vi "Create Reference Maps.vi"(8 "error in (no error)":errorcluster, 10 "RT Target":bool, 11 "LabVIEW Build Script in":refnum<class "LabVIEW Build Script.lvclass">) -> (0 "error out":errorcluster, 3 "LabVIEW Build Script out":refnum<class "LabVIEW Build Script.lvclass">)   [LabVIEW 2021, in "LabVIEW Build Script.lvclass"]
uses:
  LabVIEW Build Script.lvclass
  LabVIEW Build Script.lvclass/LabVIEW Build Script.ctl
  <vilib>/CIF Foundation/CIF LabVIEW Scripting/LV Scripting/LV Scripting Utilities.lvlib
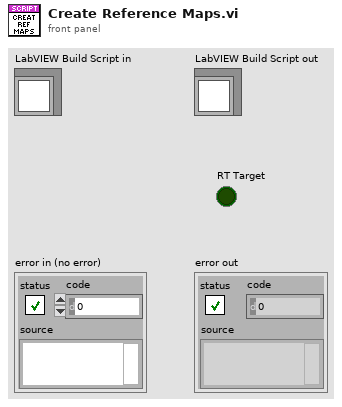
[diagram p1: front panel]
types:
  T1 = typedef "LV Scripting Utilities.lvlib/Target References.ctl" = cluster{"Target Reference":refnum<vi>, "VI References":refnum<vi>[], "Library References":refnum<vi>[], "Build References":refnum<vi>[]}
  T2 = typedef "LV Scripting Utilities.lvlib/BuildSpec Map.ctl" = map{string, refnum<vi>}
  T3 = typedef "LV Scripting Utilities.lvlib/Library Map.ctl" = map{string, refnum<vi>}
  T4 = typedef "LV Scripting Utilities.lvlib/VI Map.ctl" = map{string, refnum<vi>}
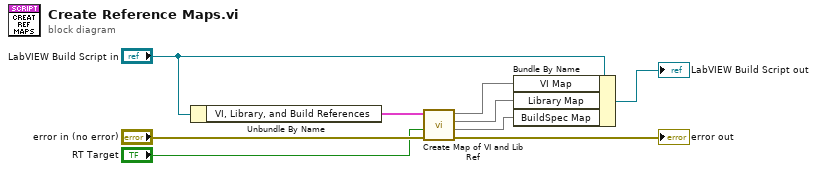
[diagram p0: block diagram]
diagram:
  n1 = Unbundle By Name("LabVIEW Build Script in") -> ("VI, Library, and Build References"=w7:T1[])
  n2 = call <vilib>:"Create Map of VI and Lib Ref.vi"("error in"="error in (no error)", "RT Target"="RT Target", "VI, Library, and Build References"=w7) -> ("error out"=→"error out":errorcluster, "BuildSpec Map"=w3:T2, "Library Map"=w1:T3, "VI Map"=w2:T4)  [unwired: 5 in]
  n3 = Bundle By Name(cluster="LabVIEW Build Script in", "VI Map"=w2, "Library Map"=w1, "BuildSpec Map"=w3) -> (→"LabVIEW Build Script out":refnum<class "LabVIEW Build Script.lvclass">)
